vi "CreateVirtualChannels.vi"(8 "error in (no error)":errorcluster, 9 "data in":T1, 11 "virtual channel config in":T5) -> (0 "error out":errorcluster, 1 "data out":T1, 3 "virtual channel config out":T5)   [LabVIEW 2017, in "McsaVirtualChannel.lvlib"]
uses:
  <vilib>/addons/InsightCM/Devices/Shared/Mcsa/McsaVirtualChannel/McsaVirtualChannel.lvlib
  <vilib>/addons/InsightCM/Devices/Shared/Mcsa/McsaVirtualChannel/controls/Config.ctl
  <vilib>/addons/InsightCM/Devices/Shared/Mcsa/McsaVirtualChannel/controls/VirtualChannelGroup.ctl
  <vilib>/addons/InsightCM/Devices/Shared/Mcsa/McsaVirtualChannel/controls/VirtualChannel.ctl
  <vilib>/addons/InsightCM/Devices/Shared/Common/DataFlow/controls/Data.ctl
  <vilib>/addons/InsightCM/Utilities/DataAccessors/controls/wfmSGL_DVR.ctl
  <vilib>/addons/PointValueMap/controls/PointMap.ctl
  <vilib>/addons/InsightCM/Devices/Shared/Common/DataFlow/controls/Type.ctl
  <vilib>/addons/PointValueMap/PointValueMap.lvlib
  <vilib>/addons/InsightCM/Devices/Shared/Common/DataFlow/DataFlow.lvlib
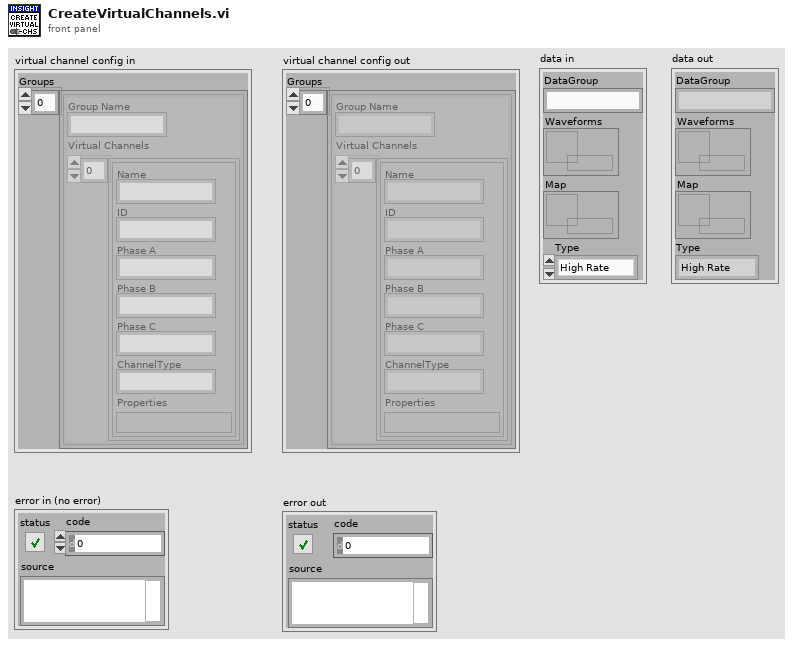
[diagram p1: front panel]
types:
  T1 = typedef "DataFlow.lvlib/Data.ctl" = cluster{"DataGroup":string, "Waveforms":T2, "Map":T3, "Type":T4}
  T2 = typedef "wfmSGL_DVR.ctl" = refnum<data-value>
  T3 = typedef "PointValueMap.lvlib/PointMap.ctl" = refnum<data-value>
  T4 = typedef "DataFlow.lvlib/Type.ctl" = enum16{"High Rate", "Low Rate", "Burst Mode"}
  T5 = typedef "McsaVirtualChannel.lvlib/Config.ctl" = cluster{"Groups":T6[]}
  T6 = typedef "McsaVirtualChannel.lvlib/VirtualChannelGroup.ctl" = cluster{"Group Name":string, "Virtual Channels":T7[]}
  T7 = typedef "McsaVirtualChannel.lvlib/VirtualChannel.ctl" = cluster{"Name":string, "ID":string, "Phase A":string, "Phase B":string, "Phase C":string, "ChannelType":string, "Properties":variant}
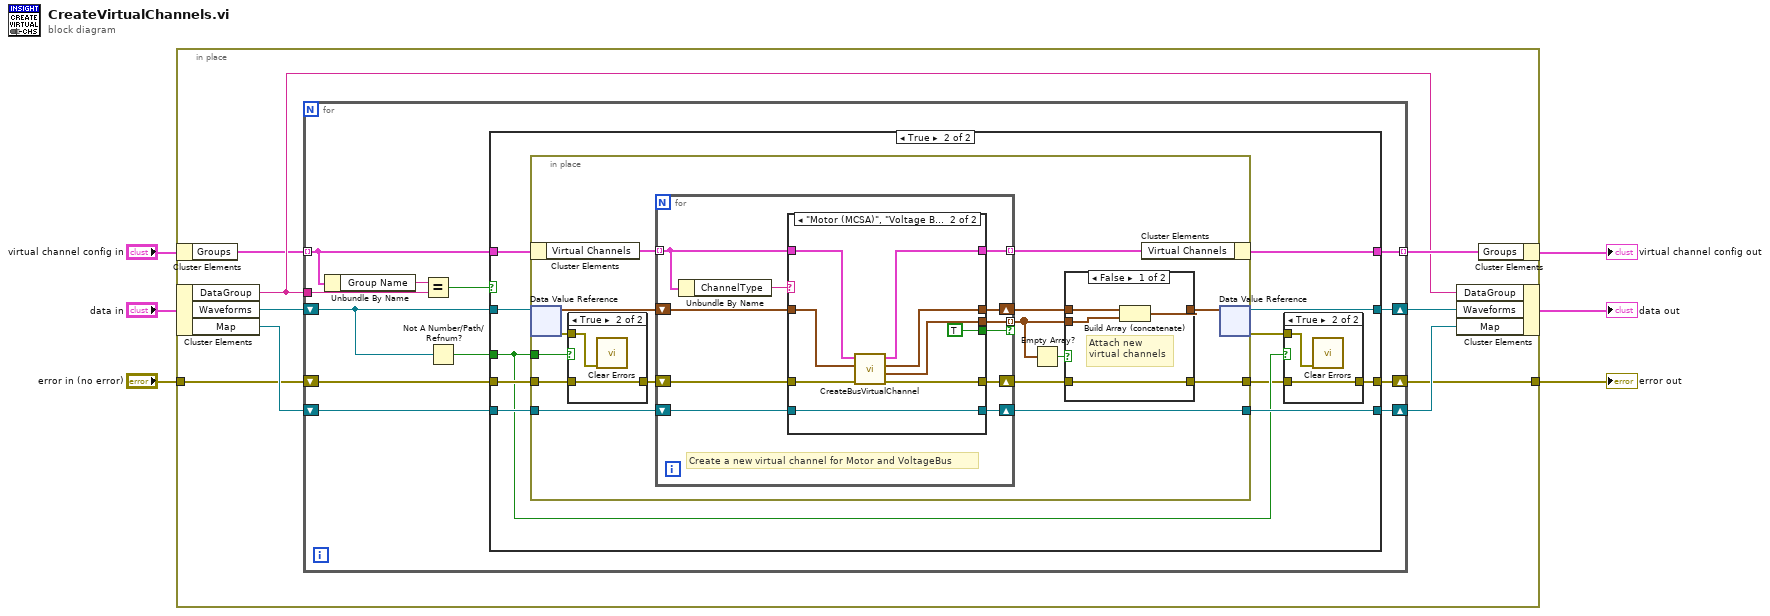
[diagram p0: block diagram]
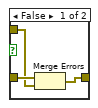
[diagram p3: hidden frame]
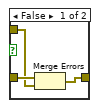
[diagram p5: hidden frame]
diagram:
  n1 = in-place {
    in-place-border: "error in (no error)" -> [w12]
    in-place-border: [w8] -> w1
    n2 = in-place-cluster #1("virtual channel config in") -> ("Groups"=w7:T6[])
    n3 = in-place-cluster #2("data in") -> ("DataGroup"=w9:string, "Waveforms"=w14:T2, "Map"=w13:T3)
    n4 = for {
      tunnel: w7 -> [w25] mode=indexing
      tunnel: w9 -> [w26]
      tunnel: [w22] -> w15 mode=indexing
      shift-right: [w20] -> w10
      shift-left: w13 -> [w24]
      shift-right: [w21] -> w8
      shift-left: w12 -> [w23]
      shift-right: [w19] -> w11
      shift-left: w14 -> [w18]
      n5 = Unbundle By Name(w25) -> ("Group Name"=w27:string)
      n6 = Equal?(x=w27, y=w26) -> (x = y?=w17:bool)
      n7 = Not A Number/Path/Refnum?(number/path/refnum=w18) -> (NaN/Path/Refnum?=w16:bool)
      n8 = case shown="True" w17 {
        tunnel: w25 -> [w31 w40]
        tunnel: w18 -> [w29 w38]
        tunnel: w24 -> [w28 w42]
        tunnel: w23 -> [w30 w41]
        tunnel: [w31 w39] -> w22
        tunnel: [w30 w32] -> w21
        tunnel: [w28 w37] -> w20
        tunnel: [w29 w36] -> w19
        tunnel: w16 -> [_ w34]
        frame False {
        }
        frame True {
          n9 = in-place {
            in-place-border: w42 -> [w62]
            in-place-border: w41 -> [w55]
            in-place-border: [w50] -> w33
            in-place-border: [w58] -> w37
            in-place-border: w34 -> [w57]
            n10 = in-place-cluster #3(w40) -> ("Virtual Channels"=w61:T7[])
            n11 = in-place-dvr #4(w38) -> (w59:waveform(sgl)[], w56:errorcluster)
            n12 = case shown="True" w57 {
              tunnel: w56 -> [w69 w73]
              tunnel: w55 -> [w70 w72]
              tunnel: [w71 w72] -> w54
              frame False {
                n13 = Merge Errors(w70, w69) -> (w71:errorcluster)
              }
              frame True {
                n14 = call <vilib>:"Clear Errors.vi"("error in (no error)"=w73) -> ()  [unwired: 5 in, 2 out]
              }
            }
            n15 = for {
              tunnel: w61 -> [w80] mode=indexing
              tunnel: [w81] -> w60 mode=indexing
              shift-right: [w77] -> w58
              shift-left: w62 -> [w78]
              shift-right: [w79] -> w53
              shift-left: w59 -> [w83]
              shift-right: [w76] -> w51
              shift-left: w54 -> [w84]
              tunnel: [w75] -> w48 mode=indexing if=w74
              # "Create a new virtual channel for Motor and VoltageBus"
              n16 = Unbundle By Name(w80) -> ("ChannelType"=w82:string)
              n17 = case shown="\"Motor (MCSA)\", \"Voltage Bus\"" w82 {
                tunnel: w84 -> [w87 w96]
                tunnel: w83 -> [w85 w93]
                tunnel: [w87 w95] -> w76
                tunnel: [w88 w94] -> w81
                tunnel: w80 -> [w88 w97]
                tunnel: [w85 w91] -> w79
                tunnel: [w86 w90] -> w77
                tunnel: w78 -> [w86 w90]
                tunnel: [_ w89] -> w75
                tunnel: [_ TRUE] -> w74
                frame Default {
                }
                frame "Motor (MCSA)", "Voltage Bus" {
                  n18 = call <vilib>:"CreateBusVirtualChannel.vi"("error in (no error)"=w96, "Wfm Data in"=w93, "Virtual Channel in"=w97) -> ("error out"=w95:errorcluster, "Created Bus Channel"=w89:waveform(sgl), "Wfm Data out"=w91:waveform(sgl)[], "Virtual Channel out"=w94:T7)  [unwired: 5 in]
                }
              }
            }
            n19 = Empty Array?(array=w48) -> (empty?=w49:bool)
            n20 = case shown="False" w49 {
              tunnel: [w63 w67] -> w50
              tunnel: w51 -> [w63 w67]
              tunnel: w48 -> [w64 _]
              tunnel: w53 -> [w66 w68]
              tunnel: [w65 w68] -> w52
              frame False {
                # "Attach new\nvirtual channels"
                n21 = Build Array (concatenate)(w66, w64) -> (w65:waveform(sgl)[])
              }
              frame True {
              }
            }
            n22 = in-place-cluster #3("Virtual Channels"=w60) -> (w39:T6)
            n23 = in-place-dvr #4(w52) -> (w36:T2, w35:errorcluster)
          }
          n24 = case shown="True" w34 {
            tunnel: w35 -> [w43 w47]
            tunnel: w33 -> [w44 w46]
            tunnel: [w45 w46] -> w32
            frame False {
              n25 = Merge Errors(w44, w43) -> (w45:errorcluster)
            }
            frame True {
              n26 = call <vilib>:"Clear Errors.vi"("error in (no error)"=w47) -> ()  [unwired: 5 in, 2 out]
            }
          }
        }
      }
    }
    n27 = in-place-cluster #2("DataGroup"=w9, "Waveforms"=w11, "Map"=w10) -> (→"data out":T1)
    n28 = in-place-cluster #1("Groups"=w15) -> (→"virtual channel config out":T5)
  }
  "error out" <- w1
